vi "9205 Read 5.vi"(8 "error in":errorcluster, 11 "Module Config Selector":i16) -> (0 "error out":errorcluster, 3 "Data Array":sgl[](array[numeric]))   [LabVIEW 2015]
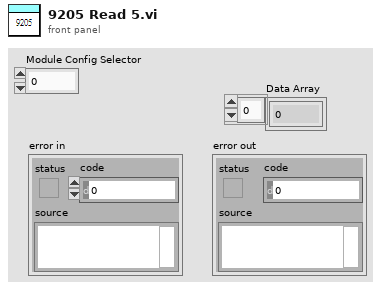
[diagram p1: front panel]
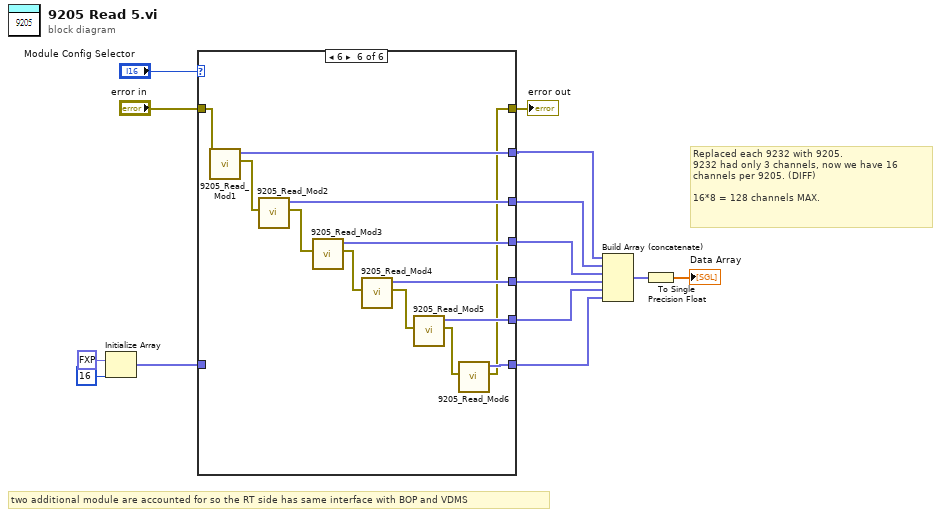
[diagram p0: block diagram]
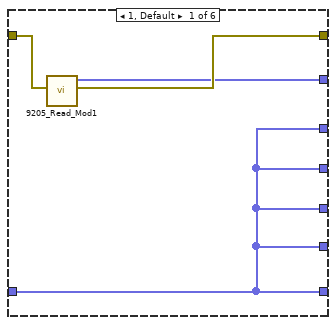
[diagram p2: hidden frame]
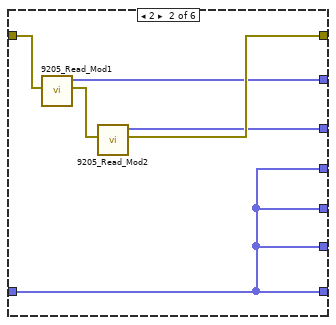
[diagram p3: hidden frame]
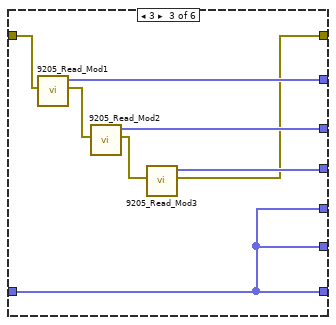
[diagram p4: hidden frame]
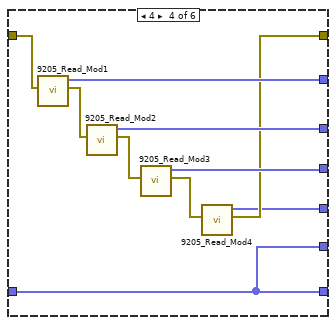
[diagram p5: hidden frame]
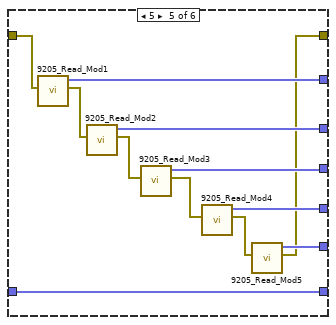
[diagram p6: hidden frame]
diagram:
  # "Replaced each 9232 with 9205.\n9232 had only 3 channels, now we have 16\nchannels per 9205. (DIFF)\n\n16*8 = 128 channels MAX."
  # "two additional module are accounted for so the RT side has same interface with BOP and VDMS"
  n1 = Initialize Array(fxp<+/-,26,5> 0.0 ("Mod1/AI0"), 16 ("dimension size")) -> (w4:fxp<+/-,26,5>[])
  n2 = case shown="6" "Module Config Selector" {
    tunnel: "error in" -> [w17 w23 w31 w42 w54 w67]
    tunnel: [w16 w21 w25 w35 w43 w55] -> w13
    tunnel: [w18 w24 w27 w38 w50 w63] -> w11
    tunnel: [w15 w20 w29 w40 w52 w65] -> w10
    tunnel: [w18 w19 w28 w39 w51 w64] -> w9
    tunnel: [w18 w24 w32 w33 w46 w60] -> w8
    tunnel: [w18 w24 w32 w34 w45 w59] -> w7
    tunnel: [w18 w24 w32 w34 w47 w57] -> w6
    tunnel: w4 -> [w18 w24 w32 w34 w47 _]
    frame 1, Default {
      n3 = call "9205_Read_Mod1.vi"("error in"=w17) -> ("error out"=w16:errorcluster, "data out"=w15:fxp<+/-,26,5>[])  [unwired: 9 in]
    }
    frame 2 {
      n4 = call "9205_Read_Mod1.vi"("error in"=w23) -> ("error out"=w22:errorcluster, "data out"=w20:fxp<+/-,26,5>[])  [unwired: 9 in]
      n5 = call "9205_Read_Mod2.vi"("error in"=w22) -> ("error out"=w21:errorcluster, "data out"=w19:fxp<+/-,26,5>[])  [unwired: 9 in]
    }
    frame 3 {
      n6 = call "9205_Read_Mod1.vi"("error in"=w31) -> ("error out"=w30:errorcluster, "data out"=w29:fxp<+/-,26,5>[])  [unwired: 9 in]
      n7 = call "9205_Read_Mod2.vi"("error in"=w30) -> ("error out"=w26:errorcluster, "data out"=w28:fxp<+/-,26,5>[])  [unwired: 9 in]
      n8 = call "9205_Read_Mod3.vi"("error in"=w26) -> ("error out"=w25:errorcluster, "data out"=w27:fxp<+/-,26,5>[])  [unwired: 9 in]
    }
    frame 4 {
      n9 = call "9205_Read_Mod1.vi"("error in"=w42) -> ("error out"=w41:errorcluster, "data out"=w40:fxp<+/-,26,5>[])  [unwired: 9 in]
      n10 = call "9205_Read_Mod2.vi"("error in"=w41) -> ("error out"=w37:errorcluster, "data out"=w39:fxp<+/-,26,5>[])  [unwired: 9 in]
      n11 = call "9205_Read_Mod3.vi"("error in"=w37) -> ("error out"=w36:errorcluster, "data out"=w38:fxp<+/-,26,5>[])  [unwired: 9 in]
      n12 = call "9205_Read_Mod4.vi"("error in"=w36) -> ("error out"=w35:errorcluster, "data out"=w33:fxp<+/-,26,5>[])  [unwired: 9 in]
    }
    frame 5 {
      n13 = call "9205_Read_Mod1.vi"("error in"=w54) -> ("error out"=w53:errorcluster, "data out"=w52:fxp<+/-,26,5>[])  [unwired: 9 in]
      n14 = call "9205_Read_Mod2.vi"("error in"=w53) -> ("error out"=w49:errorcluster, "data out"=w51:fxp<+/-,26,5>[])  [unwired: 9 in]
      n15 = call "9205_Read_Mod3.vi"("error in"=w49) -> ("error out"=w48:errorcluster, "data out"=w50:fxp<+/-,26,5>[])  [unwired: 9 in]
      n16 = call "9205_Read_Mod4.vi"("error in"=w48) -> ("error out"=w44:errorcluster, "data out"=w46:fxp<+/-,26,5>[])  [unwired: 9 in]
      n17 = call "9205_Read_Mod5.vi"("error in"=w44) -> ("error out"=w43:errorcluster, "data out"=w45:fxp<+/-,26,5>[])  [unwired: 9 in]
    }
    frame 6 {
      n18 = call "9205_Read_Mod1.vi"("error in"=w67) -> ("error out"=w66:errorcluster, "data out"=w65:fxp<+/-,26,5>[])  [unwired: 9 in]
      n19 = call "9205_Read_Mod2.vi"("error in"=w66) -> ("error out"=w62:errorcluster, "data out"=w64:fxp<+/-,26,5>[])  [unwired: 9 in]
      n20 = call "9205_Read_Mod3.vi"("error in"=w62) -> ("error out"=w61:errorcluster, "data out"=w63:fxp<+/-,26,5>[])  [unwired: 9 in]
      n21 = call "9205_Read_Mod4.vi"("error in"=w61) -> ("error out"=w58:errorcluster, "data out"=w60:fxp<+/-,26,5>[])  [unwired: 9 in]
      n22 = call "9205_Read_Mod5.vi"("error in"=w58) -> ("error out"=w56:errorcluster, "data out"=w59:fxp<+/-,26,5>[])  [unwired: 9 in]
      n23 = call "9205_Read_Mod6.vi"("error in"=w56) -> ("error out"=w55:errorcluster, "data out"=w57:fxp<+/-,26,5>[])  [unwired: 9 in]
    }
  }
  "error out" <- w13
  n24 = Build Array (concatenate)(w10, w9, w11, w8, w7, w6) -> (w2:fxp<+/-,26,5>[])
  n25 = To Single Precision Float(number=w2) -> (single precision float=→"Data Array":sgl[])
